vi "xlsx_to_JSON.vi"(7 "user.xls path":path=path "C:/Users/Mogroup-3/Desktop/AutoChem_test/user.xls", 8 "error in (no error)":errorcluster, 9 "Python version":string="3.11", 10 "experiment_no":i32, 11 "worker_ID":i32) -> (0 "error out":errorcluster, 3 "return value":string)   [LabVIEW 2020]
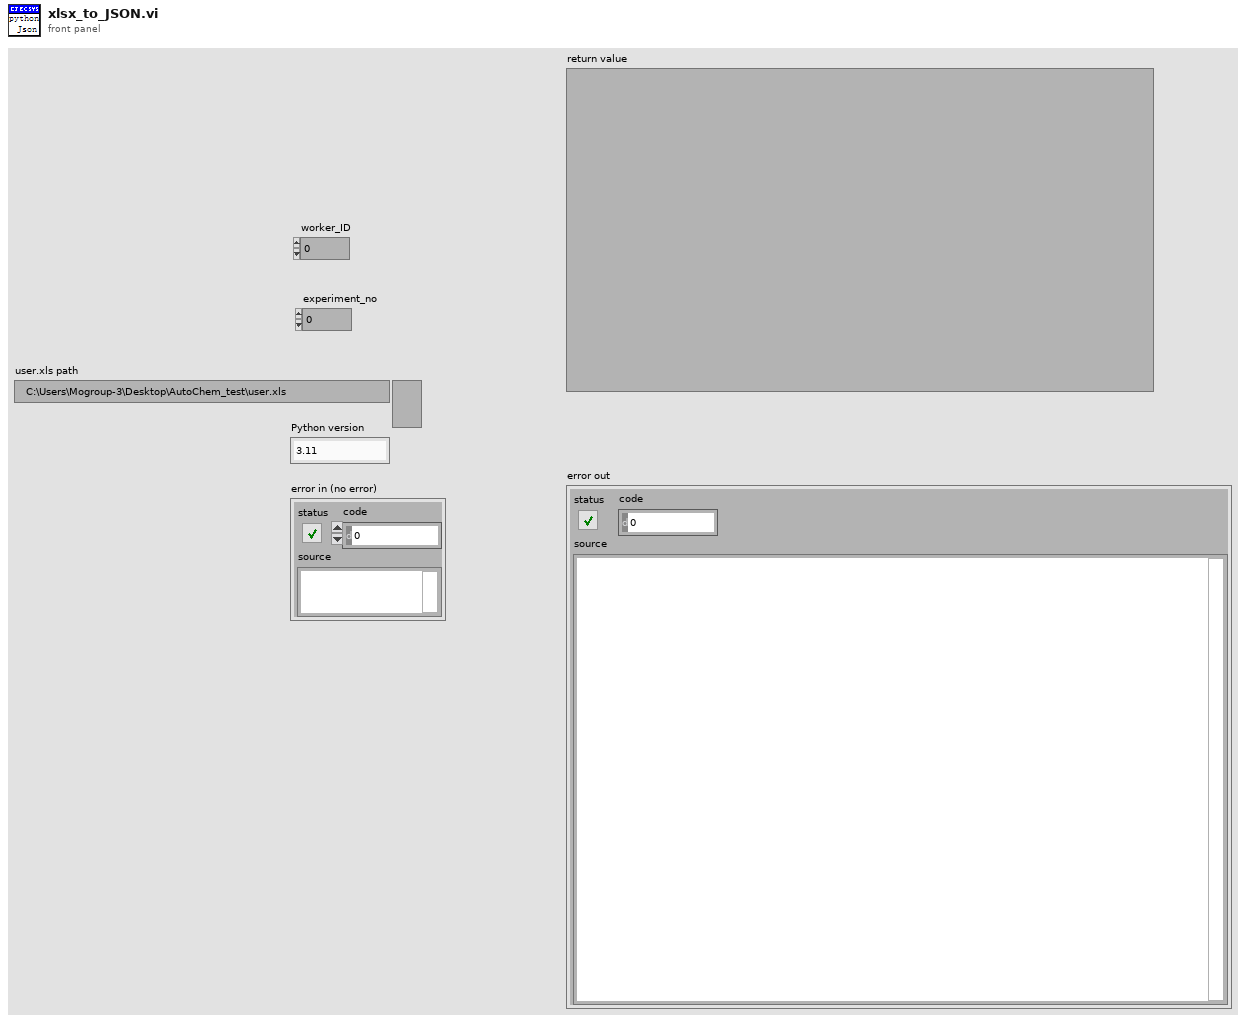
[diagram p1: front panel]
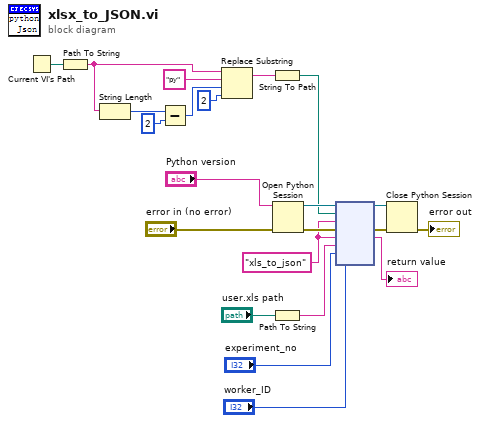
[diagram p0: block diagram]
diagram:
  w3 = "xls_to_json" ("function name")
  n1 = Current VI's Path() -> (path=w15:path)
  n2 = Path To String(path=w15) -> (string=w14:string)
  n3 = String Length(string=w14) -> (length=w11:i32)
  n4 = Subtract(x=w11, y=2) -> (x-y=w10:i32)
  n5 = Replace Substring(2:2 ("length (len. of substring)"), 3:w10, 4:"py" ("substring (\"\")"), 5:w14) -> (1:w8:string)  [unwired: 1 out]
  n6 = String To Path(string=w8) -> (path=w7:path)
  n7 = Path To String(path="user.xls path") -> (string=w6:string)
  n8 = Open Python Session(python version="Python version", 3:"error in (no error)") -> (session out=w21:refnum<k35>, error out=w18:errorcluster)  [unwired: 1 in]
  n9 = node(w21, w7, w3, w18, w3, w6, "experiment_no", "worker_ID") -> (w20:refnum<k35>, w19:errorcluster, →"return value":string)  [unwired: 3 in, 2 out]
  n10 = Close Python Session(session in=w20, error in=w19) -> (11:→"error out":errorcluster)
